vi "N_pulses_modified.vi"() -> ()   [LabVIEW 2015]
uses:
  <vilib>/MakerHub/LINX/Public/Peripherals/Digital/Digital Write N Chans.vi
  <vilib>/MakerHub/LINX/Public/Peripherals/Analog/Analog Read 1 Chan.vi
  <vilib>/MakerHub/LINX/Private/Local IO/LinxDigitalWrite.vi
  <vilib>/MakerHub/LINX/Public/Utilities/Check Channel.vi
  <vilib>/MakerHub/LINX/Public/Peripherals/Analog/Analog Read N Chans.vi
  <vilib>/MakerHub/LINX/Private/Local IO/LinxAnalogRead.vi
  <vilib>/MakerHub/LINX/Public/Utilities/Open Serial.vi
  <vilib>/MakerHub/LINX/Private/Utilties/Generate Error.vi
  <vilib>/MakerHub/LINX/LMH-LINX.lvlib
panel:
  in  "time post":u32
  in  "number of pulses":i32
  in  "low delay":u32
  in  "peak delay":u32
  out "Ref":dbl(graph)
  in  "LED":refnum<visa-resource-name>="N/A"
  out "3":dbl(graph)
  out "2":dbl(graph)
  out "4":dbl(graph)
  out "1":dbl(graph)
  out "pos":dbl
  in  "milliseconds to wait":u32
  in  "time pre":u32
  in  "Serial Port Analog":refnum<visa-resource-name>="N/A"
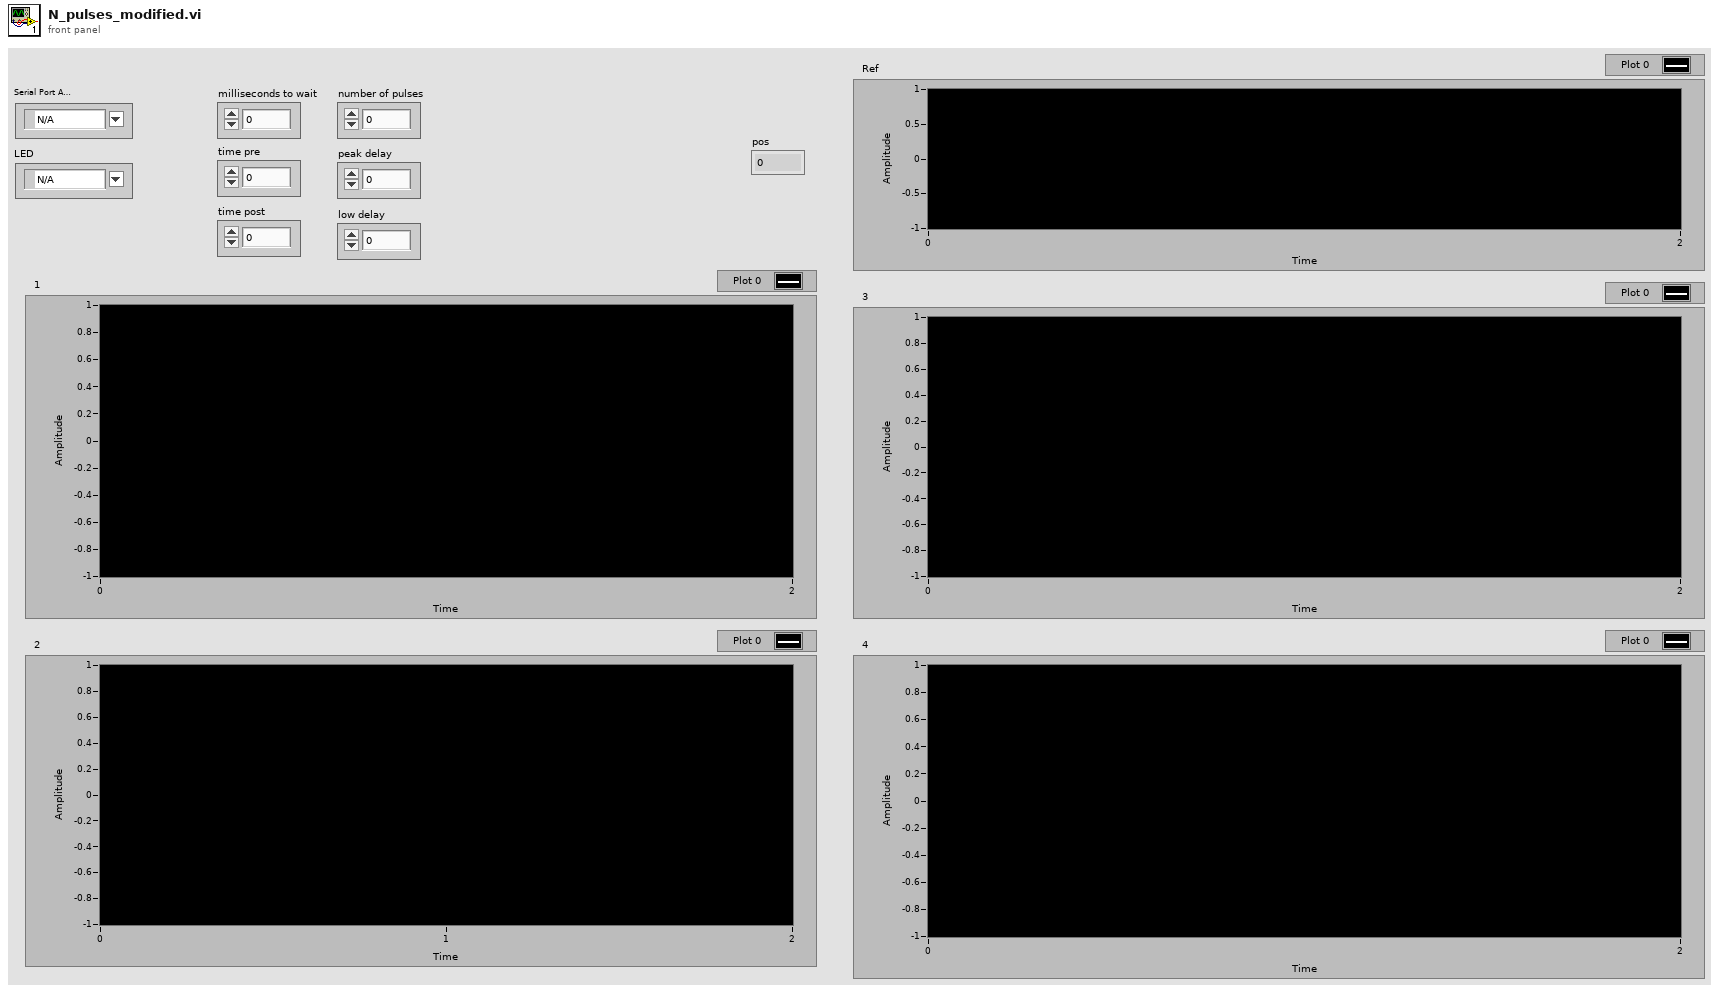
[diagram p1: front panel]
types:
  T1 = typedef "LMH-LINX.lvlib/LINX Ref.ctl" = cluster{"IO":T2, "Interface":T3, "LINX Device Config":T4}
  T2 = typedef "LMH-LINX.lvlib/Platform.ctl" = enum16{"Remote", "Local"}
  T3 = typedef "LMH-LINX.lvlib/Interface.ctl" = enum16{"Serial", "TCP"}
  T4 = typedef "LMH-LINX.lvlib/Device.lvlib/LINX Device Config.ctl" = cluster{"Interface":T3, "COM Port":refnum<visa-resource-name>, "TCP Configuration":T5, "Device Family":u8, "Device ID":u8, "Device Name":string, "TCP Ref":refnum<k5>, "Channels":T6}
  T5 = typedef "LMH-LINX.lvlib/Device.lvlib/TCP Config.ctl" = cluster{"IP Address":string, "Port":u16}
  T6 = typedef "LMH-LINX.lvlib/Channels.ctl" = cluster{"DI":u8[], "DO":u8[], "AI":u8[], "AO":u8[], "PWM":u8[], "QE":u8[], "UART":u8[], "I2C 2":u8[], "SPI":u8[], "CAN":u8[], "Servo":u8[], "AI Ref (V)":dbl, "AI Resolution (Bits)":u8, "AO Ref (V)":dbl, "AO Resolution (Bits)":u8}
  T7 = enum16{"open", "replace", "create", "open or create", "replace or create", "replace or create with confirmation"}
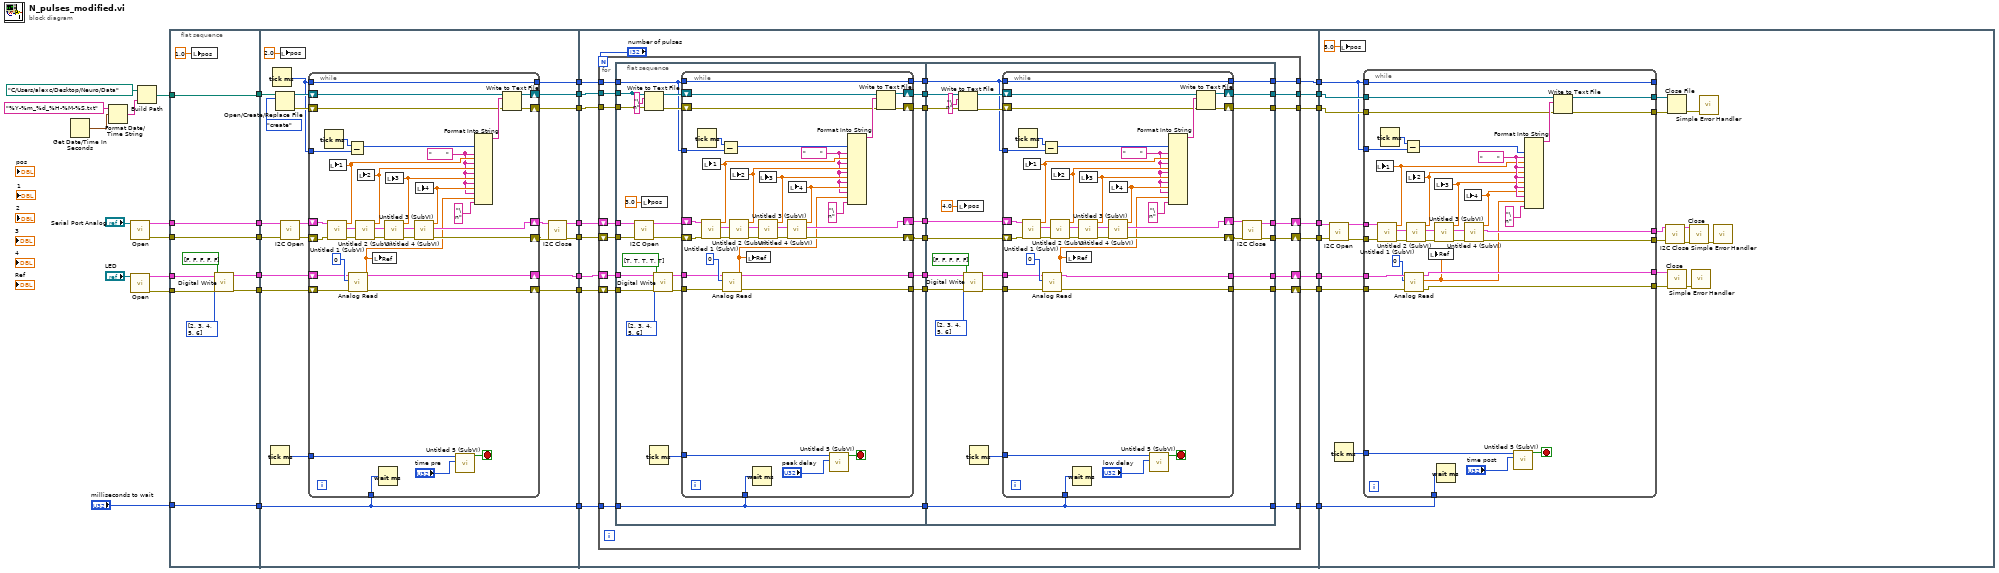
[diagram p0: block diagram]
diagram:
  n1 = Get Date/Time In Seconds() -> (seconds since 1Jan1904=w12:timestamp)
  n2 = Format Date/Time String(time format string (%c)="%Y-%m_%d_%H-%M-%S.txt", seconds (now)=w12) -> (date/time string=w14:string)  [unwired: 1 in]
  n3 = call-poly <vilib>:"Open.vi"("Serial Port"="Serial Port Analog") -> ("Error Out"=w18:errorcluster, "LINX Resource"=w19:T1)  [unwired: 8 in, 1 out]
  n4 = call-poly <vilib>:"Open.vi"("Serial Port"="LED") -> ("Error Out"=w9:errorcluster, "LINX Resource"=w10:T1)  [unwired: 8 in, 1 out]
  n5 = Build Path(base path=path "C:/Users/alexc/Desktop/Neuro/Data", name or relative path=w14) -> (appended path=w11:path)
  n6 = flat-sequence {
    tunnel: [w42] -> w34
    tunnel: [w41] -> w33
    tunnel: [w40] -> w30
    tunnel: [w35] -> w21
    tunnel: w19 -> [w42]
    tunnel: w18 -> [w41]
    tunnel: w11 -> [w40]
    tunnel: w10 -> [w39]
    tunnel: w9 -> [w38]
    tunnel: [w37] -> w8
    tunnel: [w36] -> w7
    tunnel: "milliseconds to wait" -> [w35]
    tunnel: w34 -> [w68]
    tunnel: w33 -> [w67]
    tunnel: [w66] -> w32
    tunnel: [w65] -> w31
    tunnel: w30 -> [w64]
    tunnel: [w60] -> w29
    tunnel: [w59] -> w28
    tunnel: [w57] -> w27
    tunnel: w21 -> [w55]
    tunnel: [w55] -> w20
    tunnel: w8 -> [w49]
    tunnel: w7 -> [w48]
    tunnel: [w47] -> w6
    tunnel: [w46] -> w1
    tunnel: [w110] -> w26
    tunnel: [w115] -> w25
    tunnel: [w109] -> w24
    tunnel: [w106] -> w23
    tunnel: [w104] -> w22
    tunnel: w20 -> [w116]
    tunnel: w27 -> [w108]
    tunnel: w28 -> [w105]
    tunnel: w29 -> [w107]
    tunnel: w31 -> [w118]
    tunnel: w32 -> [w119]
    tunnel: w6 -> [w120]
    tunnel: [w114] -> w4
    tunnel: [w113] -> w3
    tunnel: [w112] -> w2
    tunnel: w1 -> [w111]
    tunnel: w22 -> [w280]
    tunnel: w23 -> [w281]
    tunnel: w24 -> [w267]
    tunnel: w25 -> [w285]
    tunnel: w26 -> [w289]
    tunnel: w4 -> [w284]
    tunnel: w3 -> [w271]
    tunnel: w2 -> [w270]
    frame #0 {
      n7 = local write "pos"(1.0 ("pos")) -> ()
      n8 = call-poly <vilib>:"Digital Write.vi"("Error In"=w38, "Values"=bool[] [FALSE, FALSE, FALSE, FALSE, FALSE], "DO Channels"=u8[] [2, 3, 4, 5, 6], "LINX Resource"=w39) -> ("Error Out"=w36:errorcluster, "LINX Resource"=w37:T1)  [unwired: 6 in]
    }
    frame #1 {
      n9 = Tick Count (ms)() -> (millisecond timer value=w56:u32)
      n10 = Tick Count (ms)() -> (millisecond timer value=w58:u32)
      n11 = Open/Create/Replace File(file path (use dialog)=w64, operation (0:open)=T7."create") -> (refnum out=w62:refnum<file>, error out=w61:errorcluster)  [unwired: 4 in, 1 out]
      n12 = local write "pos"(2.0 ("pos")) -> ()
      n13 = call <vilib>:"I2C Open.vi"("Error In"=w67, "LINX Resource"=w68) -> ("Error Out"=w53:errorcluster, "LINX Resource"=w54:T1)  [unwired: 8 in]
      n14 = while {
        tunnel: w58 -> [w96]
        shift-right: [w92] -> w60
        shift-left: w62 -> [w94]
        shift-right: [w91] -> w59
        shift-left: w61 -> [w93]
        tunnel: [w90] -> w57
        tunnel: w58 -> [w90]
        tunnel: w56 -> [w89]
        tunnel: w55 -> [w71]
        shift-right: [w86] -> w52
        shift-left: w54 -> [w88]
        shift-right: [w85] -> w51
        shift-left: w53 -> [w87]
        shift-right: [w70] -> w47
        shift-left: w49 -> [w74]
        shift-right: [w69] -> w46
        shift-left: w48 -> [w73]
        stop <- w72 stop-if-true
        w78 = "       "
        n15 = Tick Count (ms)() -> (millisecond timer value=w97:u32)
        n16 = call "Untitled 1 (SubVI).vi"("error in (no error)"=w87, "LINX Resource in"=w88) -> ("error out"=w102:errorcluster, "LINX Resource out"=w103:T1, "Numeric"=w83:dbl)  [unwired: 7 in]
        n17 = local write "1"(w83) -> ()
        n18 = Subtract(x=w97, y=w96) -> (x-y=w79:u32)
        n19 = call-poly <vilib>:"Analog Read.vi"("Error In"=w73, "Analog Channel"=u8 0, "LINX Resource"=w74) -> ("Error Out"=w69:errorcluster, "Voltage"=w75:dbl, "LINX Resource"=w70:T1)  [unwired: 5 in, 1 out]
        n20 = call "Untitled 2 (SubVI).vi"("error in (no error)"=w102, "LINX Resource in"=w103) -> ("error out"=w101:errorcluster, "LINX Resource"=w100:T1, "Numeric"=w82:dbl)  [unwired: 7 in]
        n21 = local write "2"(w82) -> ()
        n22 = local write "Ref"(w75) -> ()
        n23 = Wait (ms)(milliseconds to wait=w71) -> ()  [unwired: 1 out]
        n24 = call "Untitled 3 (SubVI).vi"("error in (no error)"=w101, "LINX Resource in"=w100) -> ("error out"=w98:errorcluster, "LINX Resource out"=w99:T1, "Numeric"=w81:dbl)  [unwired: 7 in]
        n25 = local write "3"(w81) -> ()
        n26 = call "Untitled 4 (SubVI).vi"("error in (no error)"=w98, "LINX Resource in"=w99) -> ("error out"=w85:errorcluster, "LINX Resource"=w86:T1, "Numeric"=w84:dbl)  [unwired: 7 in]
        n27 = local write "4"(w84) -> ()
        n28 = call "Untitled 5 (SubVI).vi"("time_1"="time pre", "millisecond timer value"=w89) -> ("Boolean"=w72:bool)  [unwired: 9 in]
        n29 = Format Into String(w79, w78, w83, w78, w82, w78, w81, w78, w84, w78, w75, "\n") -> (resulting string=w95:string)  [unwired: 3 in, 1 out]
        n30 = Write to Text File(file (use dialog)=w94, text=w95, error in=w93) -> (refnum out=w92:refnum<file>, error out=w91:errorcluster)  [unwired: 1 in, 1 out]
      }
      n31 = call <vilib>:"I2C Close.vi"("Error In"=w51, "LINX Resource"=w52) -> ("Error Out"=w65:errorcluster, "LINX Resource"=w66:T1)  [unwired: 8 in]
    }
    frame #2 {
      n32 = for {
        N: "number of pulses" -> [_]
        tunnel: w116 -> [w134]
        tunnel: [w131] -> w114
        shift-right: [w127] -> w110
        shift-left: w119 -> [w143]
        shift-right: [w132] -> w115
        shift-left: w118 -> [w142]
        shift-right: [w130] -> w113
        shift-left: w120 -> [w144]
        shift-right: [w129] -> w112
        shift-left: w111 -> [w128]
        tunnel: [w126] -> w109
        tunnel: w108 -> [w125]
        tunnel: w107 -> [w124]
        tunnel: [w123] -> w106
        tunnel: w105 -> [w122]
        tunnel: [w121] -> w104
        n33 = flat-sequence {
          tunnel: w144 -> [w165]
          tunnel: [w145] -> _
          tunnel: w122 -> [w162]
          tunnel: w143 -> [w155]
          tunnel: w142 -> [w154]
          tunnel: w125 -> [w151]
          tunnel: [w169] -> w141
          tunnel: [w168] -> w140
          tunnel: [w164] -> w139
          tunnel: [w163] -> w138
          tunnel: [w159] -> w137
          tunnel: [w158] -> w136
          tunnel: [w150] -> w135
          tunnel: w134 -> [w147]
          tunnel: [w147] -> w133
          tunnel: w128 -> [w146]
          tunnel: w124 -> [w145]
          tunnel: w141 -> [w224]
          tunnel: w140 -> [w223]
          tunnel: w139 -> [w218]
          tunnel: w138 -> [w217]
          tunnel: w137 -> [w220]
          tunnel: w136 -> [w219]
          tunnel: w135 -> [w216]
          tunnel: w133 -> [w208]
          tunnel: [w213] -> w126
          tunnel: [w212] -> w123
          tunnel: [w211] -> w121
          tunnel: [w210] -> w127
          tunnel: [w209] -> w132
          tunnel: [w208] -> w131
          tunnel: [w207] -> w130
          tunnel: [w206] -> w129
          frame #0 {
            n34 = call <vilib>:"I2C Open.vi"("Error In"=w154, "LINX Resource"=w155) -> ("Error Out"=w152:errorcluster, "LINX Resource"=w153:T1)  [unwired: 8 in]
            n35 = local write "pos"(3.0 ("pos")) -> ()
            n36 = Write to Text File(file (use dialog)=w145, text="\n", error in=w162) -> (refnum out=w161:refnum<file>, error out=w160:errorcluster)  [unwired: 1 in, 1 out]
            n37 = Tick Count (ms)() -> (millisecond timer value=w148:u32)
            n38 = call-poly <vilib>:"Digital Write.vi"("Error In"=w146, "Values"=bool[] [TRUE, TRUE, TRUE, TRUE, TRUE], "DO Channels"=u8[] [2, 3, 4, 5, 6], "LINX Resource"=w165) -> ("Error Out"=w157:errorcluster, "LINX Resource"=w156:T1)  [unwired: 6 in]
            n39 = while {
              tunnel: w151 -> [w198]
              shift-right: [w194] -> w164
              shift-left: w161 -> [w196]
              shift-right: [w193] -> w163
              shift-left: w160 -> [w195]
              tunnel: [w192] -> w150
              tunnel: w151 -> [w192]
              tunnel: w148 -> [w191]
              tunnel: w147 -> [w173]
              shift-right: [w188] -> w169
              shift-left: w153 -> [w190]
              shift-right: [w187] -> w168
              shift-left: w152 -> [w189]
              tunnel: w156 -> [w176]
              tunnel: w157 -> [w175]
              tunnel: [w172] -> w159
              tunnel: [w171] -> w158
              stop <- w174 stop-if-true
              w180 = "       "
              n40 = Tick Count (ms)() -> (millisecond timer value=w199:u32)
              n41 = call "Untitled 1 (SubVI).vi"("error in (no error)"=w189, "LINX Resource in"=w190) -> ("error out"=w204:errorcluster, "LINX Resource out"=w205:T1, "Numeric"=w185:dbl)  [unwired: 7 in]
              n42 = local write "1"(w185) -> ()
              n43 = Subtract(x=w199, y=w198) -> (x-y=w181:u32)
              n44 = call-poly <vilib>:"Analog Read.vi"("Error In"=w175, "Analog Channel"=u8 0, "LINX Resource"=w176) -> ("Error Out"=w171:errorcluster, "Voltage"=w177:dbl, "LINX Resource"=w172:T1)  [unwired: 5 in, 1 out]
              n45 = call "Untitled 2 (SubVI).vi"("error in (no error)"=w204, "LINX Resource in"=w205) -> ("error out"=w203:errorcluster, "LINX Resource"=w202:T1, "Numeric"=w184:dbl)  [unwired: 7 in]
              n46 = local write "2"(w184) -> ()
              n47 = local write "Ref"(w177) -> ()
              n48 = Wait (ms)(milliseconds to wait=w173) -> ()  [unwired: 1 out]
              n49 = call "Untitled 3 (SubVI).vi"("error in (no error)"=w203, "LINX Resource in"=w202) -> ("error out"=w200:errorcluster, "LINX Resource out"=w201:T1, "Numeric"=w183:dbl)  [unwired: 7 in]
              n50 = local write "3"(w183) -> ()
              n51 = call "Untitled 4 (SubVI).vi"("error in (no error)"=w200, "LINX Resource in"=w201) -> ("error out"=w187:errorcluster, "LINX Resource"=w188:T1, "Numeric"=w186:dbl)  [unwired: 7 in]
              n52 = local write "4"(w186) -> ()
              n53 = call "Untitled 5 (SubVI).vi"("time_1"="peak delay", "millisecond timer value"=w191) -> ("Boolean"=w174:bool)  [unwired: 9 in]
              n54 = Format Into String(w181, w180, w185, w180, w184, w180, w183, w180, w186, w180, w177, "\n") -> (resulting string=w197:string)  [unwired: 3 in, 1 out]
              n55 = Write to Text File(file (use dialog)=w196, text=w197, error in=w195) -> (refnum out=w194:refnum<file>, error out=w193:errorcluster)  [unwired: 1 in, 1 out]
            }
          }
          frame #1 {
            n56 = local write "pos"(4.0 ("pos")) -> ()
            n57 = Write to Text File(file (use dialog)=w218, text="\n", error in=w217) -> (refnum out=w226:refnum<file>, error out=w227:errorcluster)  [unwired: 1 in, 1 out]
            n58 = call-poly <vilib>:"Digital Write.vi"("Error In"=w219, "Values"=bool[] [FALSE, FALSE, FALSE, FALSE, FALSE], "DO Channels"=u8[] [2, 3, 4, 5, 6], "LINX Resource"=w220) -> ("Error Out"=w231:errorcluster, "LINX Resource"=w230:T1)  [unwired: 6 in]
            n59 = Tick Count (ms)() -> (millisecond timer value=w214:u32)
            n60 = while {
              tunnel: w216 -> [w259]
              shift-right: [w255] -> w212
              shift-left: w226 -> [w257]
              shift-right: [w254] -> w211
              shift-left: w227 -> [w256]
              tunnel: [w253] -> w213
              tunnel: w216 -> [w253]
              tunnel: w214 -> [w252]
              tunnel: w208 -> [w234]
              shift-right: [w249] -> w222
              shift-left: w224 -> [w251]
              shift-right: [w248] -> w221
              shift-left: w223 -> [w250]
              tunnel: w230 -> [w237]
              tunnel: w231 -> [w236]
              tunnel: [w233] -> w207
              tunnel: [w232] -> w206
              stop <- w235 stop-if-true
              w241 = "       "
              n61 = Tick Count (ms)() -> (millisecond timer value=w260:u32)
              n62 = call "Untitled 1 (SubVI).vi"("error in (no error)"=w250, "LINX Resource in"=w251) -> ("error out"=w265:errorcluster, "LINX Resource out"=w266:T1, "Numeric"=w246:dbl)  [unwired: 7 in]
              n63 = local write "1"(w246) -> ()
              n64 = Subtract(x=w260, y=w259) -> (x-y=w242:u32)
              n65 = call-poly <vilib>:"Analog Read.vi"("Error In"=w236, "Analog Channel"=u8 0, "LINX Resource"=w237) -> ("Error Out"=w232:errorcluster, "Voltage"=w238:dbl, "LINX Resource"=w233:T1)  [unwired: 5 in, 1 out]
              n66 = call "Untitled 2 (SubVI).vi"("error in (no error)"=w265, "LINX Resource in"=w266) -> ("error out"=w264:errorcluster, "LINX Resource"=w263:T1, "Numeric"=w245:dbl)  [unwired: 7 in]
              n67 = local write "2"(w245) -> ()
              n68 = local write "Ref"(w238) -> ()
              n69 = Wait (ms)(milliseconds to wait=w234) -> ()  [unwired: 1 out]
              n70 = call "Untitled 3 (SubVI).vi"("error in (no error)"=w264, "LINX Resource in"=w263) -> ("error out"=w261:errorcluster, "LINX Resource out"=w262:T1, "Numeric"=w244:dbl)  [unwired: 7 in]
              n71 = local write "3"(w244) -> ()
              n72 = call "Untitled 4 (SubVI).vi"("error in (no error)"=w261, "LINX Resource in"=w262) -> ("error out"=w248:errorcluster, "LINX Resource"=w249:T1, "Numeric"=w247:dbl)  [unwired: 7 in]
              n73 = local write "4"(w247) -> ()
              n74 = call "Untitled 5 (SubVI).vi"("time_1"="low delay", "millisecond timer value"=w252) -> ("Boolean"=w235:bool)  [unwired: 9 in]
              n75 = Format Into String(w242, w241, w246, w241, w245, w241, w244, w241, w247, w241, w238, "\n") -> (resulting string=w258:string)  [unwired: 3 in, 1 out]
              n76 = Write to Text File(file (use dialog)=w257, text=w258, error in=w256) -> (refnum out=w255:refnum<file>, error out=w254:errorcluster)  [unwired: 1 in, 1 out]
            }
            n77 = call <vilib>:"I2C Close.vi"("Error In"=w221, "LINX Resource"=w222) -> ("Error Out"=w209:errorcluster, "LINX Resource"=w210:T1)  [unwired: 8 in]
          }
        }
      }
    }
    frame #3 {
      n78 = call <vilib>:"I2C Open.vi"("Error In"=w285, "LINX Resource"=w289) -> ("Error Out"=w282:errorcluster, "LINX Resource"=w283:T1)  [unwired: 8 in]
      n79 = Tick Count (ms)() -> (millisecond timer value=w279:u32)
      n80 = local write "pos"(5.0 ("pos")) -> ()
      n81 = while {
        tunnel: w284 -> [w316]
        tunnel: w283 -> [w315]
        tunnel: w282 -> [w314]
        tunnel: [w308] -> _
        tunnel: w267 -> [w308]
        tunnel: w281 -> [w307]
        tunnel: w280 -> [w306]
        tunnel: w279 -> [w305]
        tunnel: [w304] -> w278
        tunnel: [w303] -> w277
        tunnel: [w302] -> w274
        tunnel: [w301] -> w273
        tunnel: w271 -> [w300]
        tunnel: w270 -> [w299]
        tunnel: [w298] -> w269
        tunnel: [w297] -> w268
        tunnel: w267 -> [w295]
        stop <- w317 stop-if-true
        w320 = "       "
        n82 = call "Untitled 1 (SubVI).vi"("error in (no error)"=w314, "LINX Resource in"=w315) -> ("error out"=w313:errorcluster, "LINX Resource out"=w324:T1, "Numeric"=w310:dbl)  [unwired: 7 in]
        n83 = local write "1"(w310) -> ()
        n84 = Tick Count (ms)() -> (millisecond timer value=w309:u32)
        n85 = Subtract(x=w309, y=w295) -> (x-y=w294:u32)
        n86 = call-poly <vilib>:"Analog Read.vi"("Error In"=w299, "Analog Channel"=u8 0, "LINX Resource"=w300) -> ("Error Out"=w297:errorcluster, "Voltage"=w293:dbl, "LINX Resource"=w298:T1)  [unwired: 5 in, 1 out]
        n87 = call "Untitled 2 (SubVI).vi"("error in (no error)"=w313, "LINX Resource in"=w324) -> ("error out"=w312:errorcluster, "LINX Resource"=w323:T1, "Numeric"=w292:dbl)  [unwired: 7 in]
        n88 = local write "2"(w292) -> ()
        n89 = local write "Ref"(w293) -> ()
        n90 = call "Untitled 3 (SubVI).vi"("error in (no error)"=w312, "LINX Resource in"=w323) -> ("error out"=w311:errorcluster, "LINX Resource out"=w322:T1, "Numeric"=w291:dbl)  [unwired: 7 in]
        n91 = local write "3"(w291) -> ()
        n92 = Wait (ms)(milliseconds to wait=w316) -> ()  [unwired: 1 out]
        n93 = call "Untitled 4 (SubVI).vi"("error in (no error)"=w311, "LINX Resource in"=w322) -> ("error out"=w301:errorcluster, "LINX Resource"=w302:T1, "Numeric"=w290:dbl)  [unwired: 7 in]
        n94 = local write "4"(w290) -> ()
        n95 = call "Untitled 5 (SubVI).vi"("time_1"="time post", "millisecond timer value"=w305) -> ("Boolean"=w317:bool)  [unwired: 9 in]
        n96 = Format Into String(w294, w320, w310, w320, w292, w320, w291, w320, w290, w320, w293, "\n") -> (resulting string=w321:string)  [unwired: 3 in, 1 out]
        n97 = Write to Text File(file (use dialog)=w307, text=w321, error in=w306) -> (refnum out=w304:refnum<file>, error out=w303:errorcluster)  [unwired: 1 in, 1 out]
      }
      n98 = call <vilib>:"I2C Close.vi"("Error In"=w273, "LINX Resource"=w274) -> ("Error Out"=w275:errorcluster, "LINX Resource"=w276:T1)  [unwired: 8 in]
      n99 = Close File(refnum=w278, error in=w277) -> (error out=w288:errorcluster)  [unwired: 1 out]
      n100 = call <vilib>:"Close.vi"("Error In"=w268, "LINX Resource"=w269) -> ("Error Out"=w272:errorcluster)  [unwired: 9 in]
      n101 = call <vilib>:"Close.vi"("Error In"=w275, "LINX Resource"=w276) -> ("Error Out"=w287:errorcluster)  [unwired: 9 in]
      n102 = call <vilib>:"Simple Error Handler.vi"("error in (no error)"=w272) -> ()  [unwired: 4 in, 5 out]
      n103 = call <vilib>:"Simple Error Handler.vi"("error in (no error)"=w288) -> ()  [unwired: 4 in, 5 out]
      n104 = call <vilib>:"Simple Error Handler.vi"("error in (no error)"=w287) -> ()  [unwired: 4 in, 5 out]
    }
  }
